vi "Save CSV.vi"(7 "CSV Type":enum16{"Header", "Data"}(ring), 8 "error in (no error)":errorcluster, 9 "Data":variant, 10 "GlobalData":T2, 11 "file path (dialog if empty)":path) -> (0 "error out":errorcluster, 3 "new file path (Not A Path if cancelled)":path)   [LabVIEW 2024]
doc: "This VI used to create CSV file needed to save the data which include create headers and the data itself"
uses:
  controls/GlobalData.ctl
  controls/Units.ctl
  <vilib>/Utility/file.llb/Write Delimited Spreadsheet (string).vi
  <vilib>/Utility/file.llb/Write Delimited Spreadsheet (DBL).vi
  <userlib>/_OpenG.lib/lvdata/lvdata.llb/openg_variant.lvlib
panel:
  in  "Units Settings":T1={"Pressure"=enum."Pa", "Temperature"=enum."F", "Salinity"=enum."ppt", "Weight"=enum."ib"}
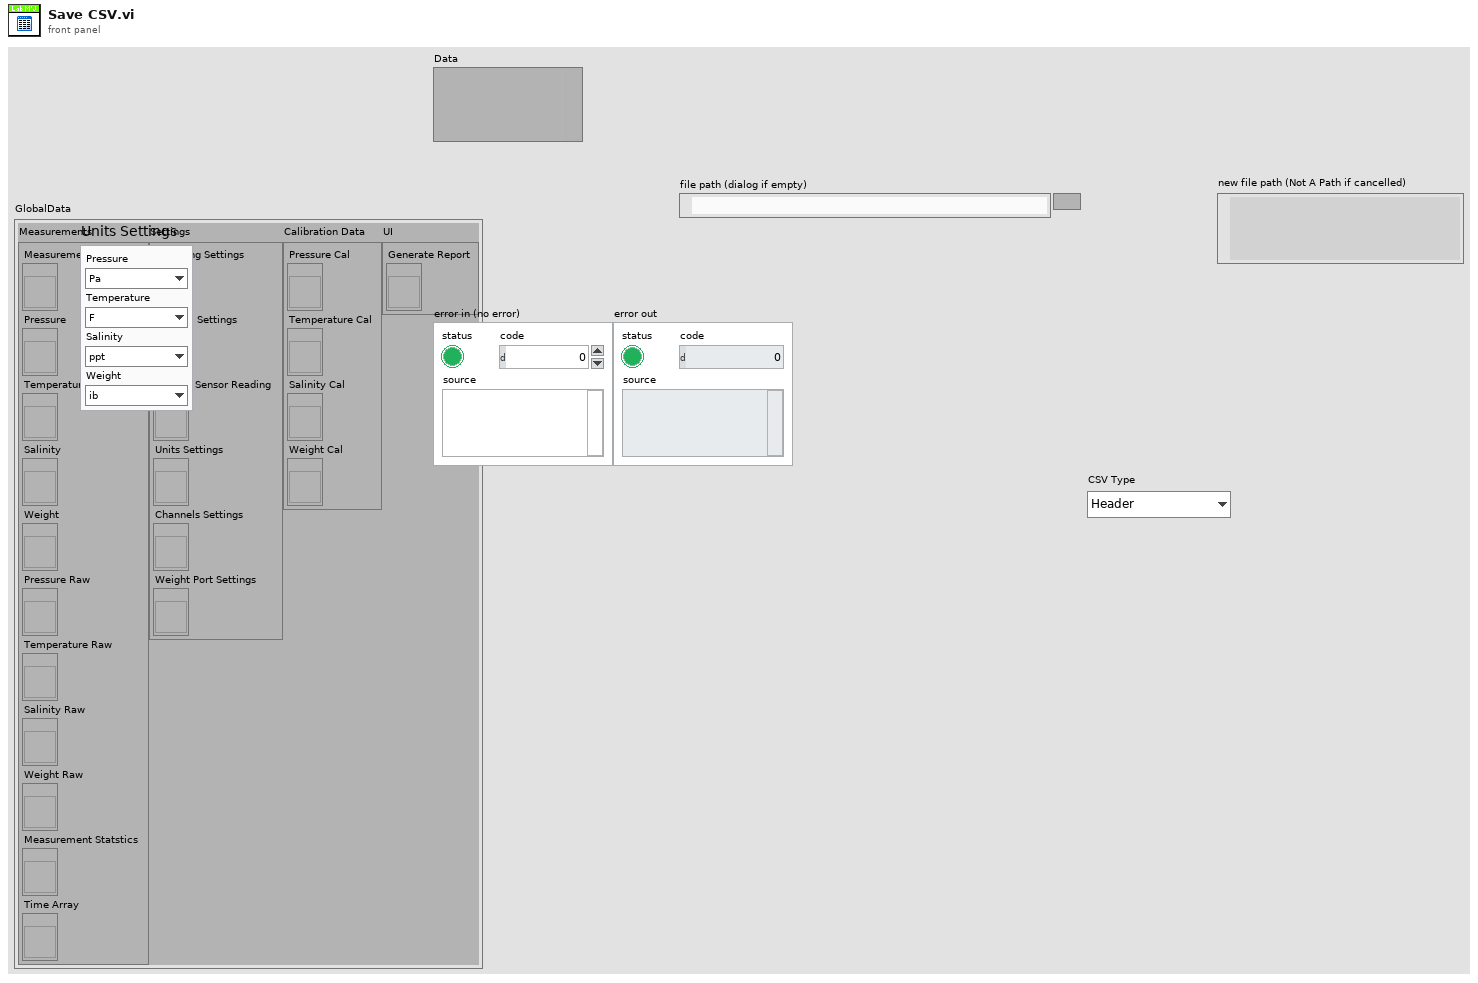
[diagram p1: front panel]
types:
  T1 = typedef "Units.ctl" = cluster{"Pressure":enum16{"PSI", "Bar", "atm", "Pa"}, "Temperature":enum16{"C", "K", "F"}, "Salinity":enum16{"ppm", "ppt", "PSU"}, "Weight":enum16{"Kg", "g", "oz", "ib"}}
  T2 = typedef "GlobalData.ctl" = cluster{"Measurements":cluster{"Measurement Graphs":refnum<vi>, "Pressure":refnum<vi>, "Temperature":refnum<vi>, "Salinity":refnum<vi>, "Weight":refnum<vi>, "Pressure Raw":refnum<vi>, "Temperature Raw":refnum<vi>, "Salinity Raw":refnum<vi>, "Weight Raw":refnum<vi>, "Measurement Statstics":refnum<vi>, "Time Array":refnum<vi>}, "Settings":cluster{"Sampling Settings":refnum<vi>, "General Settings":refnum<vi>, "Disable Sensor Reading":refnum<vi>, "Units Settings":refnum<vi>, "Channels Settings":refnum<vi>, "Weight Port Settings":refnum<vi>}, "Calibration Data":cluster{"Pressure Cal":refnum<vi>, "Temperature Cal":refnum<vi>, "Salinity Cal":refnum<vi>, "Weight Cal":refnum<vi>}, "UI":cluster{"Generate Report":refnum<vi>}}
  T3 = cluster{"Reading Time (ms)":u64, "Graph Time ":u16}
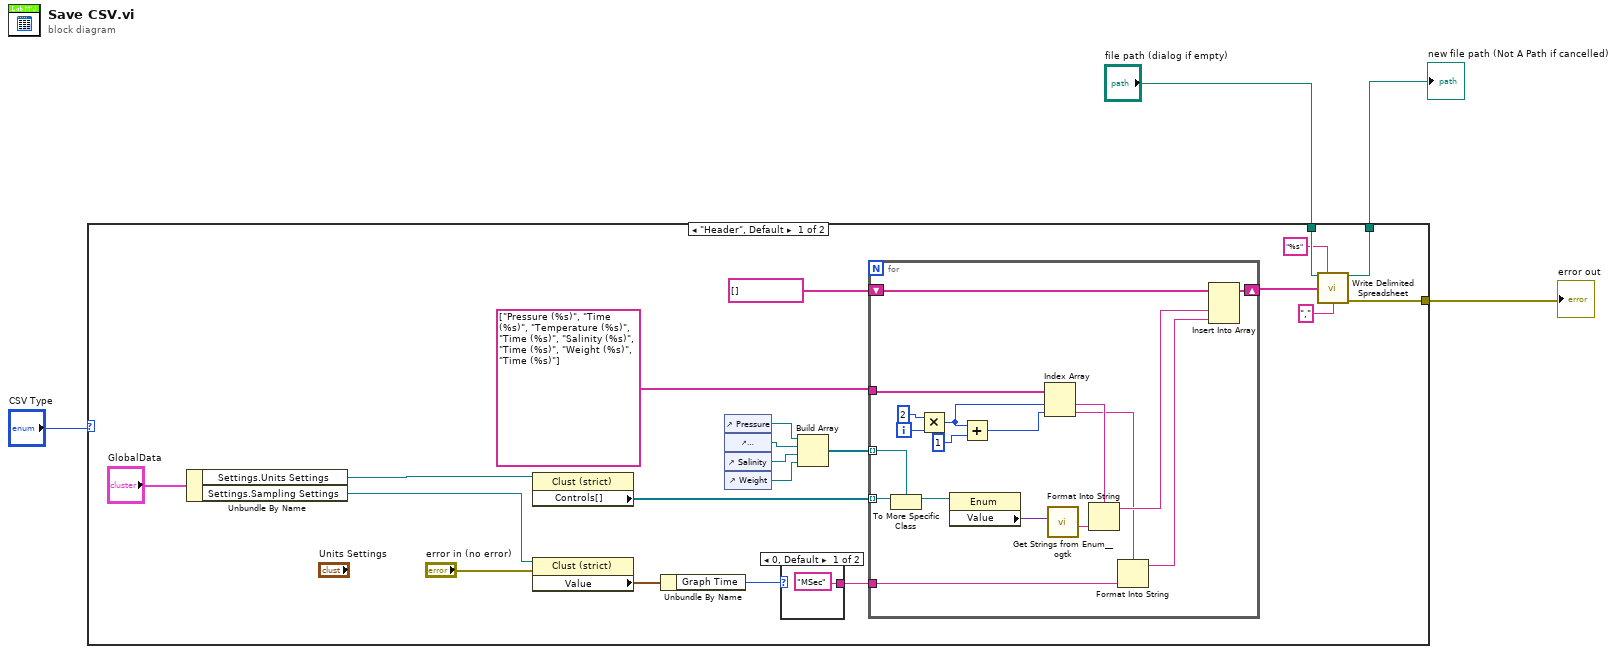
[diagram p0: block diagram]
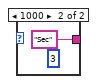
[diagram p2: hidden frame]
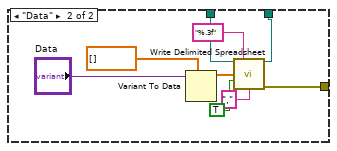
[diagram p3: hidden frame]
diagram:
  n1 = case shown="\"Header\", Default" "CSV Type" {
    tunnel: "file path (dialog if empty)" -> [w16 w50]
    tunnel: [w14 w49] -> w3
    tunnel: [w13 w48] -> w2
    frame "Header", Default {
      n2 = Unbundle By Name("GlobalData") -> ("Settings.Units Settings"=w24:refnum<vi>, "Settings.Sampling Settings"=w21:refnum<vi>)
      n3 = property on="Property Node" class="Clust (strict)"(reference=w24) -> ("Controls[]"=w23:refnum<vi>[])  [unwired: 1 in, 2 out]
      n4 = property on="Property Node" class="Clust (strict)"(reference=w21, error in="error in (no error)") -> ("Value"=w22:T3)  [unwired: 2 out]
      n5 = Unbundle By Name(w22) -> ("Graph Time"=w19:u16)
      n6 = control-ref of="Pressure"() -> (w9:refnum<vi>)
      n7 = control-ref of="Temperature"() -> (w10:refnum<vi>)
      n8 = control-ref of="Salinity"() -> (w11:refnum<vi>)
      n9 = control-ref of="Weight"() -> (w12:refnum<vi>)
      n10 = case shown="0, Default" w19 {
        tunnel: ["MSec" ("X Scale.Name Label.Text") "Sec" ("X Scale.Name Label.Text")] -> w20
        frame 0, Default {
        }
        frame 1000 {
          (unwired) u64 3 ("Reading Time (ms)")
        }
      }
      n11 = Build Array(w9, w10, w11, w12) -> (w8:refnum<vi>[])
      n12 = for {
        tunnel: w23 -> [w43] mode=indexing
        tunnel: w20 -> [w39]
        tunnel: string[] ["Pressure (%s)", "Time (%s)", "Temperature (%s)", "Time (%s)", "Salinity (%s)", "Time (%s)", "Weight (%s)", "Time (%s)"] ("channel name(s) in (Untitled)") -> [w38]
        tunnel: w8 -> [w27] mode=indexing
        shift-right: [w28] -> w15
        shift-left: string[] [] -> [w26]
        i -> [w37]
        n13 = To More Specific Class(target class=w27, reference=w43) -> (specific class reference=w42:refnum<vi>)  [unwired: 1 in, 1 out]
        n14 = Multiply(x=2, y=w37) -> (x*y=w32:i32)
        n15 = property on="Property Node" class="Enum"(reference=w42) -> ("Value"=w41:variant)  [unwired: 1 in, 2 out]
        n16 = Add(x=w32, y=1) -> (x+y=w30:i32)
        n17 = Index Array(array=w38, index #1=w32, index #2=w30) -> (element #1=w35:string, element #2=w29:string)
        n18 = call <userlib>:"Get Strings from Enum__ogtk.vi"("Enum"=w41) -> ("String Value"=w40:string)  [unwired: 7 in, 3 out]
        n19 = Format Into String(format string=w35, w40) -> (resulting string=w34:string)  [unwired: 2 in, 1 out]
        n20 = Format Into String(format string=w29, w39) -> (resulting string=w33:string)  [unwired: 2 in, 1 out]
        n21 = Insert Into Array(array=w26, new element #1=w34, new element #2=w33) -> (w28:string[])  [unwired: 1 in]
      }
      n22 = call-poly <vilib>:"Write Delimited Spreadsheet.vi"("file path (dialog if empty)"=w16, "format (%s)"="%s", "1D data"=w15, "delimiter (\\t)"="," ("delimiter (\\t)")) -> ("new file path (Not A Path if cancelled)"=w14:path, "error out"=w13:errorcluster)  [unwired: 10 in]
    }
    frame "Data" {
      n23 = Variant To Data(type=dbl[] [] ("appended array"), Variant="Data") -> (data=w54:dbl[])  [unwired: 1 in, 1 out]
      n24 = call-poly <vilib>:"Write Delimited Spreadsheet.vi"("file path (dialog if empty)"=w50, "format (%.3f)"="%.3f", "1D data"=w54, "append to file? (new file:F)"=TRUE, "delimiter (\\t)"="," ("delimiter (\\t)")) -> ("new file path (Not A Path if cancelled)"=w49:path, "error out"=w48:errorcluster)  [unwired: 9 in]
    }
  }
  "error out" <- w2
  "new file path (Not A Path if cancelled)" <- w3
